vi "init CA.vi"(7 "Command":string, 8 "error in":errorcluster, 9 "Device":u16, 10 "Card":u16, 11 "IOC":string) -> (0 "error out":errorcluster, 3 "CA out":T1)   [LabVIEW 2022 SP3]
uses:
  pectus/global/global IOC database.vi
  pectus/control/ca cluster.ctl
panel:
  out "Type":string
  out "record":string
  out "Prefix":string
  out "Ca":string
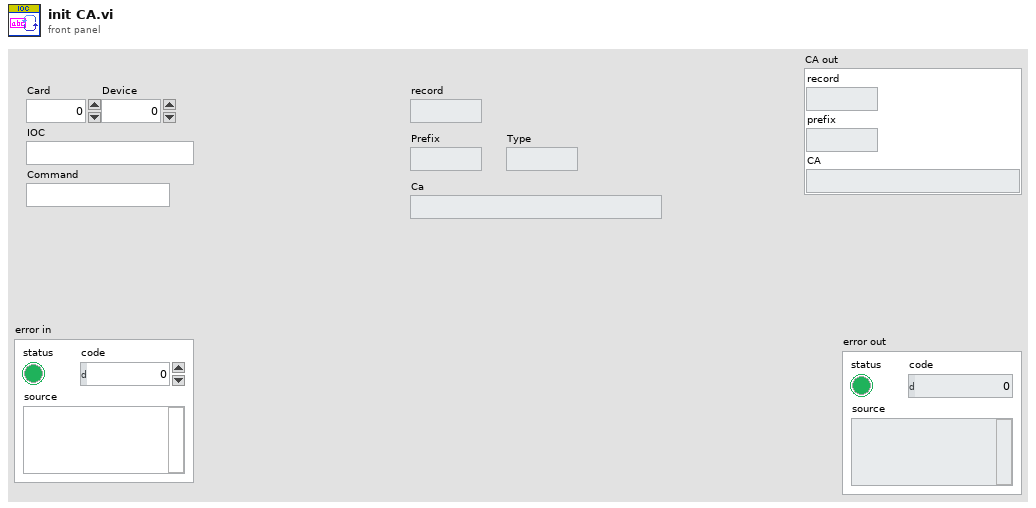
[diagram p1: front panel]
types:
  T1 = typedef "ca cluster.ctl" = cluster{"record":string, "prefix":string, "CA":string}
  T2 = typedef "epics database.ctl" = cluster{"IOC":string, "db":string, "Field Values":string[], "Values":string[][], "Type":string, "Card":u16, "Num Dev":u16}
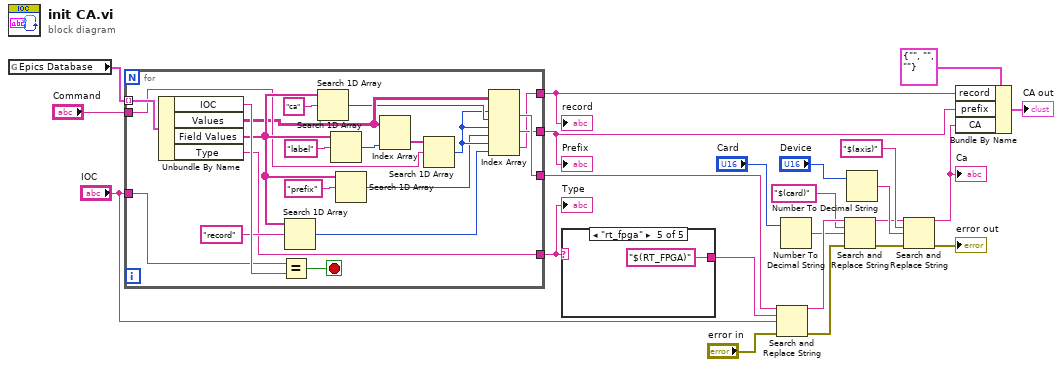
[diagram p0: block diagram]
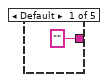
[diagram p2: hidden frame]
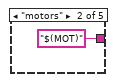
[diagram p3: hidden frame]
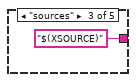
[diagram p4: hidden frame]
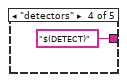
[diagram p5: hidden frame]
diagram:
  n1 = global read "global IOC database.vi" "Epics Database"() -> (w23:T2[])
  n2 = for {
    tunnel: w23 -> [w44] mode=indexing
    tunnel: "IOC" -> [w42]
    tunnel: "Command" -> [w33]
    tunnel: [w27] -> w19
    tunnel: [w26] -> w3
    tunnel: [w25] -> w4
    tunnel: [w24] -> w21
    stop <- w41 stop-if-true
    n3 = Unbundle By Name(w44) -> ("IOC"=w43:string, "Values"=w32:string[][], "Field Values"=w36:string[], "Type"=w24:string)
    n4 = Equal?(x=w42, y=w43) -> (x = y?=w41:bool)
    n5 = Search 1D Array(1D array=w36, element="record") -> (index of element=w28:i32)  [unwired: 1 in]
    n6 = Search 1D Array(1D array=w36, element="ca") -> (index of element=w31:i32)  [unwired: 1 in]
    n7 = Search 1D Array(1D array=w36, element="label") -> (index of element=w35:i32)  [unwired: 1 in]
    n8 = Search 1D Array(1D array=w36, element="prefix") -> (index of element=w29:i32)  [unwired: 1 in]
    n9 = Index Array(array=w32, index (col)=w35) -> (element=w34:string[])  [unwired: 1 in]
    n10 = Search 1D Array(1D array=w34, element=w33) -> (index of element=w30:i32)  [unwired: 1 in]
    n11 = Index Array(array=w32, index (row) #1=w30, index (col) #1=w31, index (row) #2=w30, index (col) #2=w29, index (row) #3=w30, index (col) #3=w28) -> (element #1=w27:string, element #2=w26:string, element #3=w25:string)
  }
  "Prefix" <- w3
  "record" <- w4
  "Type" <- w21
  n12 = case shown="\"rt_fpga\"" w21 {
    tunnel: ["" ("element") "$(MOT)" ("element") "$(XSOURCE)" ("element") "$(DETECT)" ("element") "$(RT_FPGA)" ("element")] -> w20
    frame Default {
    }
    frame "motors" {
    }
    frame "sources" {
    }
    frame "detectors" {
    }
    frame "rt_fpga" {
    }
  }
  n13 = Search and Replace String(input string=w19, search string=w20, replace string="IOC", error in="error in") -> (result string=w17:string, error out=w8:errorcluster)  [unwired: 4 in, 2 out]
  n14 = Number To Decimal String(number="Card") -> (decimal integer string=w14:string)  [unwired: 1 in]
  n15 = Search and Replace String(input string=w17, search string="$(card)" ("input string"), replace string=w14, error in=w8) -> (result string=w10:string, error out=w7:errorcluster)  [unwired: 4 in, 2 out]
  n16 = Number To Decimal String(number="Device") -> (decimal integer string=w13:string)  [unwired: 1 in]
  n17 = Search and Replace String(input string=w10, search string="$(axis)" ("input string"), replace string=w13, error in=w7) -> (result string=w2:string, error out=→"error out":errorcluster)  [unwired: 4 in, 2 out]
  "Ca" <- w2
  n18 = Bundle By Name(cluster=T1 {"record"="", "prefix"="", "CA"=""}, "record"=w4, "prefix"=w3, "CA"=w2) -> (→"CA out":T1)
